vi "CalculateTemperature.vi"(1 "Droptime (ms)":i32, 2 "Isotope":i32, 3 "2-D Fit Parameters":T1={"amplitude"=0.23148758679921552, "sigma_y (m)"=0.00016515813746658883, "sigma_x (m)"=0.00015948087942818507, "x offset"=74.9981011501281, "y offset"=94.78647350619177, "offset"=0.0034690691996381515, "slope x"=-4.493862455663237e-06, "slope y"=-2.2534990898103273e-06, 0.0}) -> (0 "Avg. Temp":ext)   [LabVIEW 2013]
uses:
  <vilib>/express/express arith-compare/Formula/XNode/ExpressFormulaBlockNode.xnode
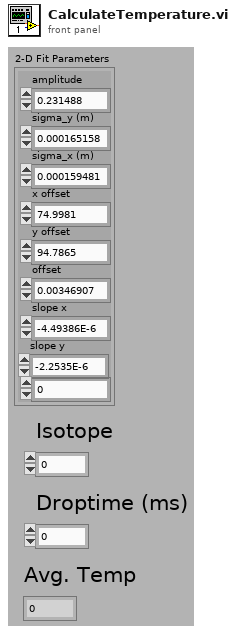
[diagram p1: front panel]
types:
  T1 = cluster{"amplitude":dbl, "sigma_y (m)":dbl, "sigma_x (m)":dbl, "x offset":dbl, "y offset":dbl, "offset":dbl, "slope x":dbl, "slope y":dbl, dbl}
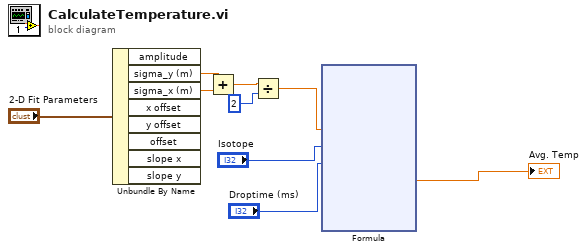
[diagram p0: block diagram]
diagram:
  n1 = Unbundle By Name("2-D Fit Parameters") -> ("sigma_y (m)"=w8:dbl, "sigma_x (m)"=w7:dbl)  [unwired: 6 out]
  n2 = Add(x=w8, y=w7) -> (x+y=w6:dbl)
  n3 = Divide(x=w6, y=2) -> (x/y=w4:dbl)
  n4 = xnode "Formula"("SigmaAvg"=w4, "Isotope"="Isotope", "Droptime"="Droptime (ms)") -> ("Result"=→"Avg. Temp":dbl)  [unwired: 1 in, 1 out]
